vi "UART.vi"(1 "Baud Rate":u32, 2 "Input":i16) -> ()   [LabVIEW 2015]
uses:
  <vilib>/rvi/Emulation/niFpgaGetClockAttributes.vi
  <vilib>/rvi/Emulation/niFpgaSctlEmulationGetInTimedLoop.vi
  <vilib>/rvi/Emulation/niFpgaEmulationReportErrorSimple.vi
  <vilib>/rvi/eio/common/nirviEmuTemplateMethod_errors.vi
  <vilib>/rvi/Emulation/niFpgaCriticalErrorInLSC.vi
  <vilib>/eio/EIONode/EIONode.xnode
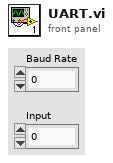
[diagram p1: front panel]
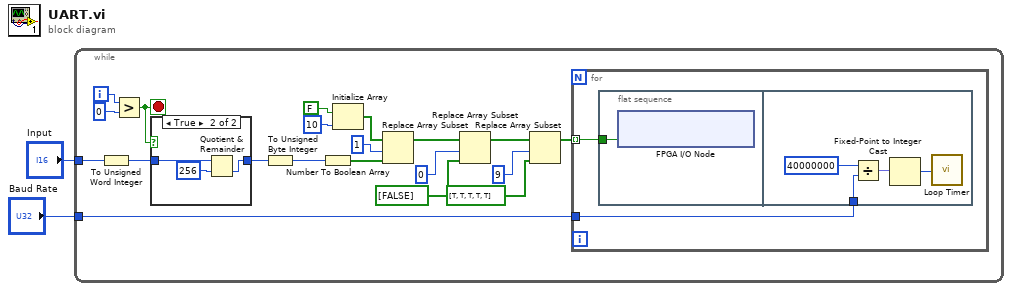
[diagram p0: block diagram]
diagram:
  n1 = while {
    tunnel: "Input" -> [w9]
    tunnel: "Baud Rate" -> [w3]
    i -> [w7]
    stop <- w4 stop-if-true
    n2 = To Unsigned Word Integer(number=w9) -> (unsigned 16bit integer=w8:u16)
    n3 = Greater?(x=w7, y=i16 0) -> (0:w4:bool)
    n4 = case shown="True" w4 {
      tunnel: [w23 w24] -> w6
      tunnel: w8 -> [w23 w26]
      frame False {
      }
      frame True {
        n5 = Quotient & Remainder(x=w26, y=u16 256) -> (floor(x/y)=w24:u16)  [unwired: 1 out]
      }
    }
    n6 = To Unsigned Byte Integer(number=w6) -> (unsigned 8bit integer=w5:u8)
    n7 = Number To Boolean Array(number=w5) -> (Boolean array=w14:bool[])
    n8 = Initialize Array(FALSE, i16 10) -> (w12:bool[])
    n9 = Replace Array Subset(array=w12, new element=w14, index=1) -> (w15:bool[])
    n10 = Replace Array Subset(array=w15, new element=bool[] [FALSE], index=0) -> (w20:bool[])
    n11 = Replace Array Subset(array=w20, new element=bool[] [TRUE, TRUE, TRUE, TRUE, TRUE], index=9) -> (w21:bool[])
    n12 = for {
      tunnel: w21 -> [w28] mode=indexing
      tunnel: w3 -> [w27]
      n13 = flat-sequence {
        tunnel: w28 -> [w29]
        tunnel: w27 -> [w30]
        frame #0 {
          n14 = xnode "FPGA I/O Node"("Connector1/DIO0"=w29) -> ()  [unwired: 1 in, 1 out]
        }
        frame #1 {
          n15 = Divide(x=40000000, y=w30) -> (x/y=w32:fxp<+/-,16,16>)
          n16 = Fixed-Point to Integer Cast(1:w32) -> (0:w31:i16)
          n17 = call "Loop Timer"("Count(Ticks)"=w31) -> ()  [unwired: 1 out]
        }
      }
    }
  }
